vi "ReadAndLoadMovie.vi"() -> ()   [LabVIEW 2015]
uses:
  <vilib>/addons/h5labview2/base/lib_path.vi
  <vilib>/addons/h5labview2/base/H5Equery.vi
  <vilib>/addons/h5labview2/attrib/H5Aread.llb/H5Aread.xnode
  <vilib>/addons/h5labview2/dataset/H5Dread.llb/H5Dread.xnode
  <vilib>/addons/h5labview2/file/H5F.lvlib
  <vilib>/addons/h5labview2/group/H5G.lvlib
  <vilib>/addons/h5labview2/space/H5S.lvlib
panel:
  in  "Frame":i32
  out "size(s)":i32
  out "dims":u32[](array[numeric])
  out "Data out":u16[](array[numeric])
  out "img_idx":u16[](array[numeric])
  out "DAQ Data":dbl[][](array[numeric])
  in  "Combo Box":string(combo)
  out "ypixels":i32
  out "xpixels":i32
  out "error out":errorcluster
  out "Object Names":string[](array[string])
  in  "Path":path
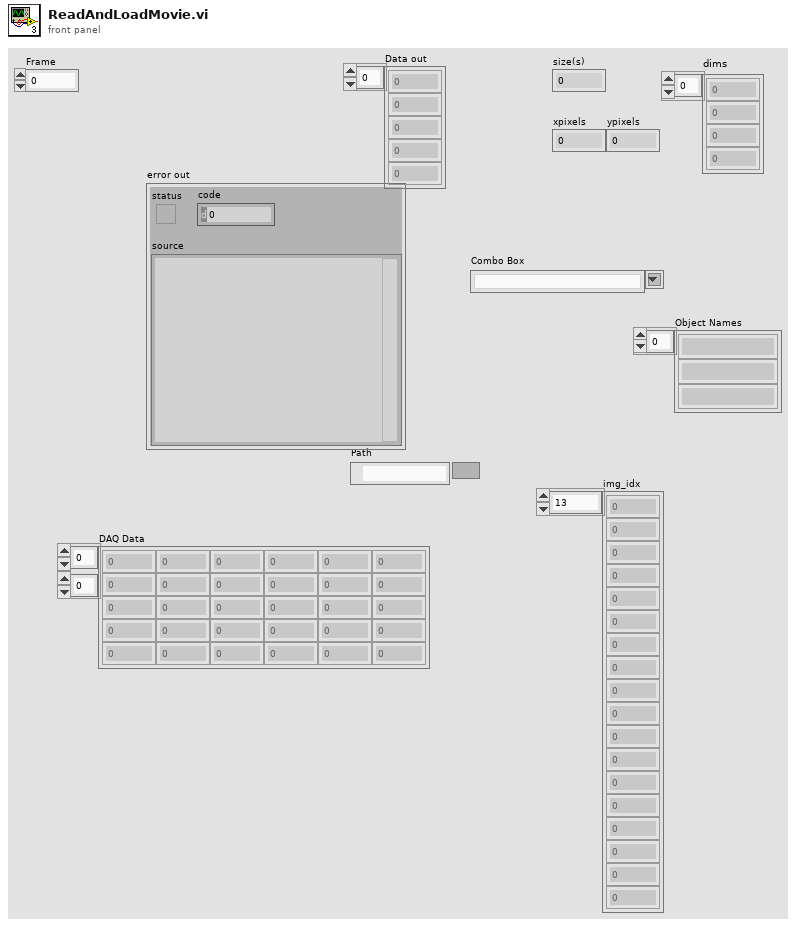
[diagram p1: front panel]
types:
  T1 = typedef "hid_t.ctl" = i32
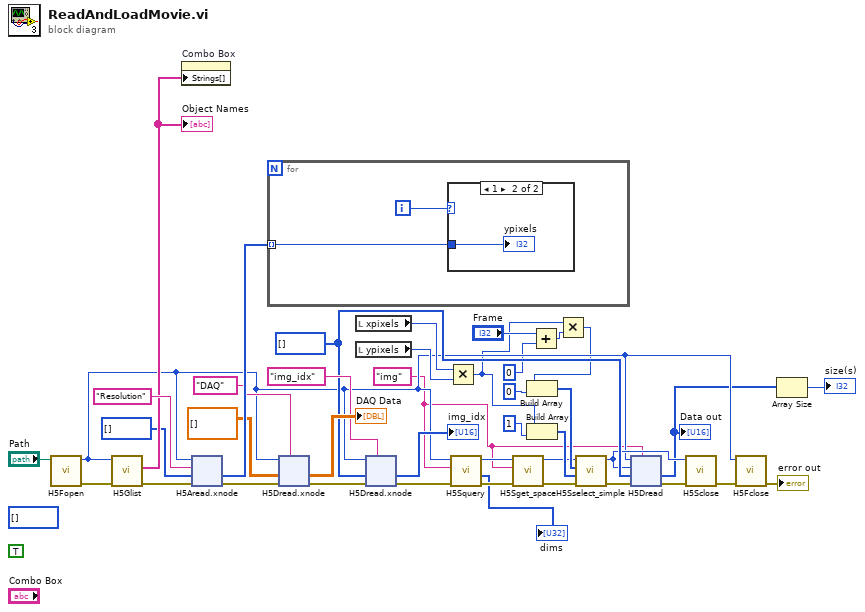
[diagram p0: block diagram]
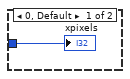
[diagram p2: hidden frame]
diagram:
  w10 = "img" ("Combo Box")
  w21 = u16[] []
  (unwired) i32[] []
  (unwired) TRUE ("Force Close (F)")
  n1 = call <vilib>:"H5Fopen.vi"("path"="Path") -> ("error out"=w40:errorcluster, "ref out"=w16:T1)  [unwired: 9 in]
  n2 = call <vilib>:"H5Glist.vi"("error in (no error)"=w40, "ref in"=w16) -> ("error out"=w37:errorcluster, "names"=w36:string[])  [unwired: 6 in, 2 out]
  "Object Names" <- w36
  n3 = property on="Combo Box" class="CmbBox"("Strings[]"=w36) -> ()  [unwired: 2 in, 2 out]
  n4 = xnode "H5Aread.xnode"("error in (no error)"=w37, "default"=i32[] [], "attrib name"="Resolution" ("name"), "ref in"=w16) -> ("error out"=w27:errorcluster, "data"=w28:i32[])  [unwired: 2 in, 2 out]
  n5 = for {
    tunnel: w28 -> [w42] mode=indexing
    i -> [w43]
    n6 = case shown="1" w43 {
      tunnel: w42 -> [w44 w45]
      frame 0, Default {
        "xpixels" <- w44
      }
      frame 1 {
        "ypixels" <- w45
      }
    }
  }
  n7 = xnode "H5Dread.xnode"("dataset name (this)"="DAQ" ("Combo Box"), "error in (no error)"=w27, "default"=dbl[][] [], "ref in"=w16) -> ("error out"=w35:errorcluster, "data"=→"DAQ Data":dbl[][])  [unwired: 2 in, 2 out]
  n8 = local read "xpixels"() -> (w32:i32)
  n9 = local read "ypixels"() -> (w31:i32)
  n10 = xnode "H5Dread.xnode"("dataset name (this)"="img_idx" ("Combo Box"), "error in (no error)"=w35, "default"=w21, "ref in"=w16) -> ("error out"=w13:errorcluster, "data"=→"img_idx":u16[])  [unwired: 2 in, 2 out]
  n11 = Multiply(x=w32, y=w31) -> (x*y=w2:i32)
  n12 = call <vilib>:"H5Squery.vi"("error in (no error)"=w13, "obj"=w10, "ref in"=w16) -> ("error out"=w12:errorcluster, "dims"=→"dims":u32[], "ref out"=w15:T1)  [unwired: 5 in, 1 out]
  n13 = call <vilib>:"H5Sget_space.vi"("error in (no error)"=w12, "obj"=w10, "ref in"=w15) -> ("error out"=w11:errorcluster, "space out"=w14:T1)  [unwired: 7 in]
  n14 = Build Array(w2, 1 ("element")) -> (w22:i32[])
  n15 = Add(x="Frame", y=0) -> (x+y=w3:i32)
  n16 = Multiply(x=w2, y=w3) -> (x*y=w1:i32)
  n17 = Build Array(w1, 0 ("element")) -> (w23:i32[])
  n18 = call <vilib>:"H5Sselect_simple.vi"("error in (no error)"=w11, "count"=w22, "start"=w23, "space in"=w14) -> ("error out"=w20:errorcluster, "space out"=w17:T1)  [unwired: 6 in]
  n19 = xnode "H5Dread"("dataset name (this)"=w10, "error in (no error)"=w20, "default"=w21, "file space"=w17, "ref in"=w16) -> ("error out"=w19:errorcluster, "data"=w7:u16[])  [unwired: 1 in, 2 out]
  "Data out" <- w7
  n20 = call <vilib>:"H5Sclose.vi"("error in (no error)"=w19, "space in"=w17) -> ("error out"=w18:errorcluster)  [unwired: 9 in]
  n21 = call <vilib>:"H5Fclose.vi"("error in (no error)"=w18, "ref"=w16) -> ("error out"=→"error out":errorcluster)  [unwired: 9 in]
  n22 = Array Size(array=w7) -> (size(s)=→"size(s)":i32)
